vi "Align to Shoot.vi"() -> (0 "Stop?":bool, 3 "Aligned?":bool)   [LabVIEW 2015]
uses:
  Robot Values.vi
  <vilib>/ptbypt/NI_PtbyPt.lvlib
panel:
  in  "Drive Motor Power":dbl=0.8 format="%#_13g"
  in  "Target Target Distance (ft)":dbl=10.0 format="%#_13g"
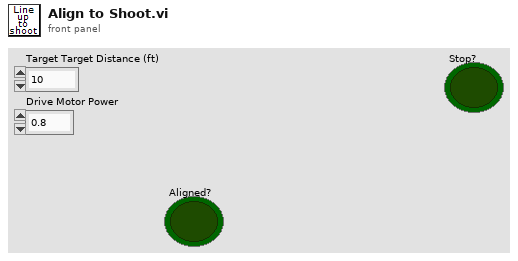
[diagram p1: front panel]
types:
  T1 = typedef "Robot Values.ctl" = cluster{"Drive Motors":cluster{"Left Motor Value":dbl, "Right Motor Value":dbl, "Left Motor Encoder":dbl, "Right Motor Encoder":dbl, "High/Low Gear":bool}, "Sensors":cluster{"Gyro Angle":dbl, "Photoeye":bool, "Ultrasonic Range":dbl, "Shooter Speed Encoder":dbl, "Accelerometer Value":dbl, "Flashlight":bool, "Target Distance":dbl, "Target X Value":dbl, "Reset Gyro?":bool}, "Arms":cluster{"Desired Arm Position":dbl, "Left Arm Encoder":dbl, "Right Arm Encoder":dbl, "Left Arm Lower Limit":bool, "Right Arm Lower Limit":bool, "Initialize Arm Position?":bool}, "Acquisition and Scoring":cluster{"Acquiring?":bool, "Current Speed":dbl, "Setpoint Speed":dbl, "Prep Wheels":bool, "Shoot":bool, "Low Eject":bool, "Reverse Shooter Wheel":bool}, "Hanging":cluster{"Pivot Arms":dbl, "PTO":bool, "Left Pivot Encoder":dbl, "Right Pivot Encoder":dbl, "Hanging Pin":bool}}
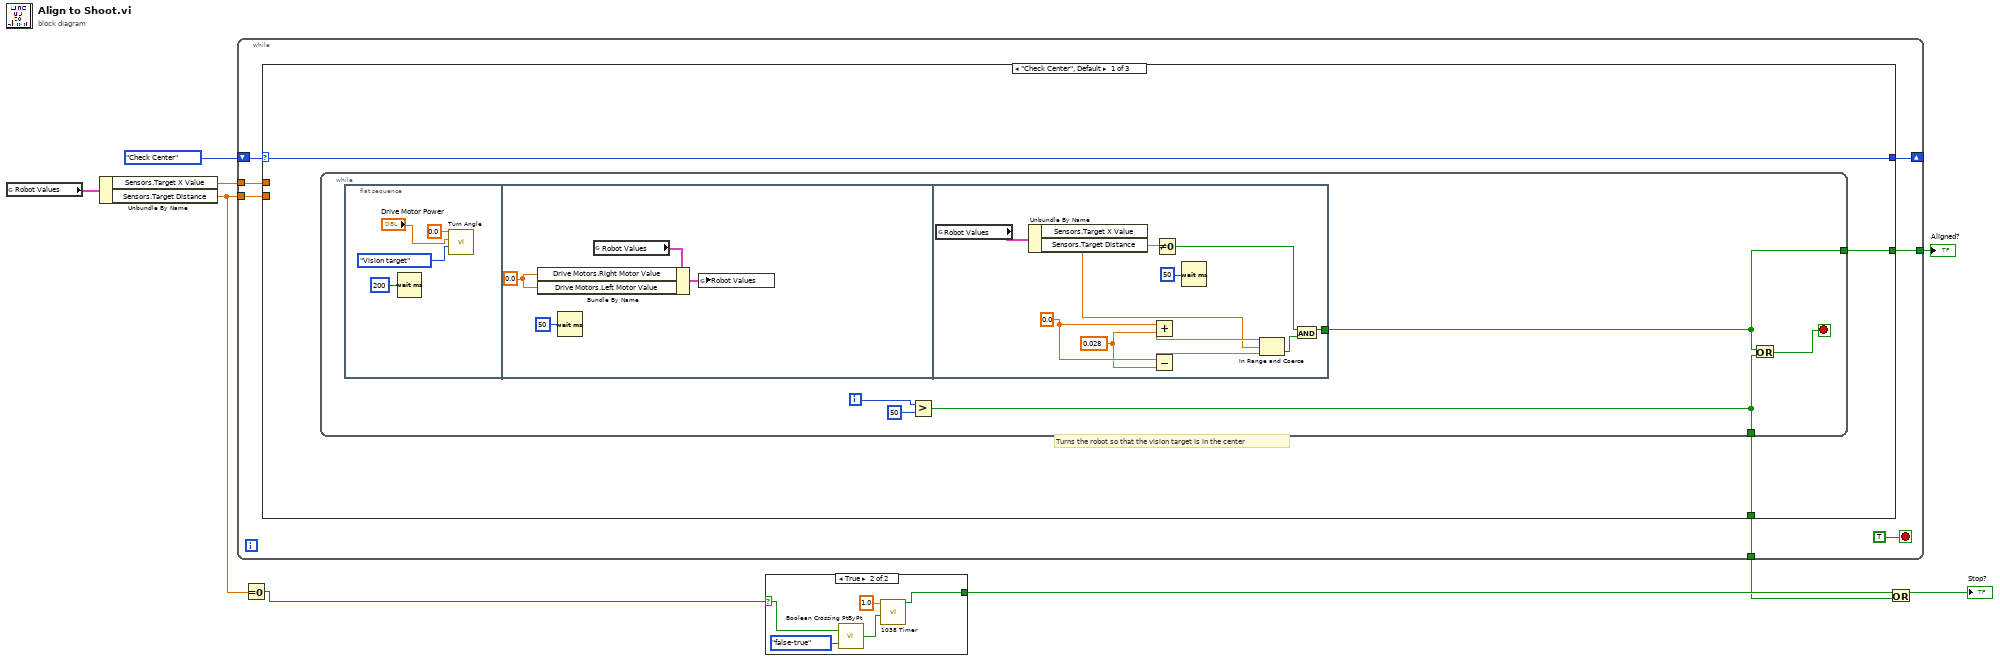
[diagram p0: block diagram]
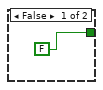
[diagram p2: hidden frame]
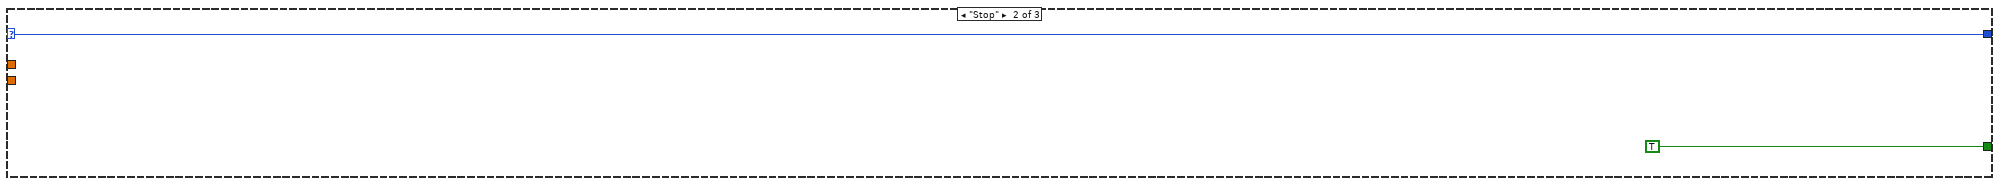
[diagram p3: hidden frame]
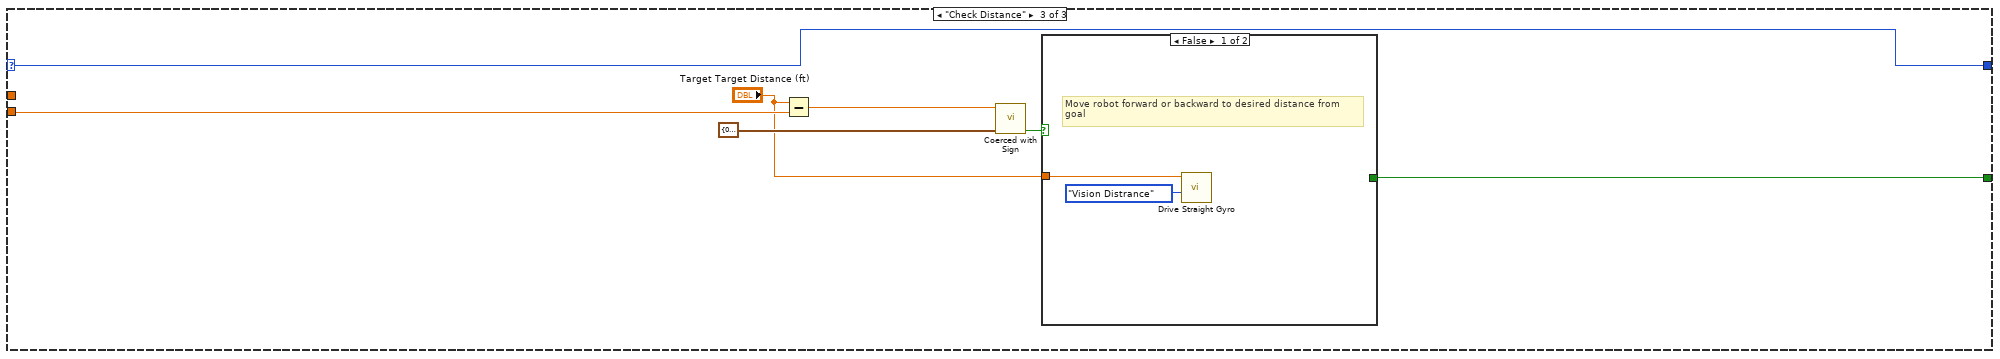
[diagram p4: hidden frame]
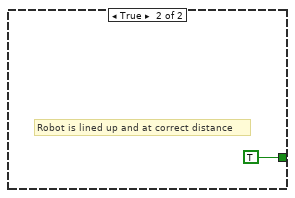
[diagram p5: hidden frame]
diagram:
  n1 = global read "Robot Values.vi" "Robot Values"() -> (w7:T1)
  n2 = Unbundle By Name(w7) -> ("Sensors.Target X Value"=w6:dbl, "Sensors.Target Distance"=w5:dbl)
  n3 = while {
    shift-right: [w13] -> _
    shift-left: enum16{"Check Center", "Stop", "Check Distance"}."Check Center" -> [w15]
    tunnel: w6 -> [w14]
    tunnel: [w12] -> w8
    tunnel: w5 -> [w11]
    tunnel: [w10] -> w1
    stop <- TRUE stop-if-true
    n4 = case shown="\"Check Center\", Default" w15 {
      selector: w15 -> [w19 w44 w46]
      tunnel: w14 -> [_ _ _]
      tunnel: [w19 w44 w46] -> w13
      tunnel: [w18 TRUE w50] -> w12
      tunnel: w11 -> [_ _ w49]
      tunnel: [w17 _ _] -> w10
      frame "Check Center", Default {
        # "Turns the robot so that the vision target is in the center"
        n5 = while {
          tunnel: [w21] -> w18
          tunnel: [w20] -> w17
          i -> [w24]
          stop <- w22 stop-if-true
          n6 = flat-sequence {
            tunnel: [w35] -> w21
            frame #0 {
              n7 = Wait (ms)(milliseconds to wait=u32 200) -> ()  [unwired: 1 out]
              n8 = call "Turn Angle.vi"("Process Variable type (Gyro)"=enum16{"Gyro", "Vision target"}."Vision target" ("Process Variable type"), "Motor Power"="Drive Motor Power", "setpoint"=0.0) -> ()  [unwired: 8 in, 1 out]
            }
            frame #1 {
              w31 = 0.0
              n9 = Wait (ms)(milliseconds to wait=u32 50) -> ()  [unwired: 1 out]
              n10 = global read "Robot Values.vi" "Robot Values"() -> (w30:T1)
              n11 = Bundle By Name(cluster=w30, "Drive Motors.Right Motor Value"=w31, "Drive Motors.Left Motor Value"=w31) -> (w29:T1)
              n12 = global write "Robot Values.vi" "Robot Values"(w29) -> ()
            }
            frame #2 {
              w40 = 0.028 ("Tolerence")
              w43 = 0.0
              n13 = global read "Robot Values.vi" "Robot Values"() -> (w39:T1)
              n14 = Unbundle By Name(w39) -> ("Sensors.Target X Value"=w38:dbl, "Sensors.Target Distance"=w36:dbl)
              n15 = Add(x=w43, y=w40) -> (x+y=w41:dbl)
              n16 = Subtract(x=w43, y=w40) -> (x-y=w42:dbl)
              n17 = Not Equal To 0?(x=w36) -> (x != 0?=w33:bool)
              n18 = Wait (ms)(milliseconds to wait=u32 50) -> ()  [unwired: 1 out]
              n19 = In Range and Coerce(upper limit=w41, x=w38, lower limit=w42) -> (In Range?=w34:bool)  [unwired: 1 out]
              n20 = And(x=w33, y=w34) -> (x .and. y?=w35:bool)
            }
          }
          n21 = Greater?(x=w24, y=50) -> (0:w20:bool)
          n22 = Or(x=w21, y=w20) -> (x .or. y?=w22:bool)
        }
      }
      frame "Stop" {
      }
      frame "Check Distance" {
        n23 = Subtract(x="Target Target Distance (ft)", y=w49) -> (x-y=w47:dbl)
        n24 = call "Coerced with Sign.vi"("Input"=w47, "Limits"=cluster{"\"Upper\"":dbl, "\"Lower\"":dbl} {"\"Upper\""=0.5, "\"Lower\""=-0.5}) -> ("In Range?"=w51:bool)  [unwired: 7 in, 1 out]
        n25 = case shown="False" w51 {
          tunnel: [_ TRUE] -> w50
          tunnel: "Target Target Distance (ft)" -> [w54 _]
          frame False {
            # "Move robot forward or backward to desired distance from\ngoal"
            n26 = call "Drive Straight Gyro.vi"("Process Variable type (Encoders)"=enum16{"Encoders", "Vision Distrance"}."Vision Distrance" ("Process Variable type"), "Distance to travel"=w54) -> ()  [unwired: 9 in, 1 out]
          }
          frame True {
            # "Robot is lined up and at correct distance"
          }
        }
      }
    }
  }
  "Aligned?" <- w8
  n27 = Equal To 0?(x=w5) -> (x = 0?=w4:bool)
  n28 = case shown="True" w4 {
    selector: w4 -> [_ w57]
    tunnel: [FALSE w60] -> w3
    frame False {
    }
    frame True {
      n29 = call <vilib>:"Boolean Crossing PtByPt.vi"("direction"=enum16{"either", "false-true", "true-false"}."false-true", "input"=w57) -> ("crossing"=w58:bool)  [unwired: 1 in]
      n30 = call "1038 Timer.vi"("Reset?"=w58, "Time Target"=1.0) -> ("Done?"=w60:bool)  [unwired: 9 in]
    }
  }
  n31 = Or(x=w3, y=w1) -> (x .or. y?=→"Stop?":bool)
